vi "Unregister Event.vi"(8 "error in (no error)":errorcluster, 9 "EventToken":refnum<class "EventToken.lvclass">, 11 "ActiveObjectEventManager in":refnum<class "EventManager.lvclass">) -> (0 "error out":errorcluster, 3 "ActiveObjectEventManager out":refnum<class "EventManager.lvclass">)   [LabVIEW 2009, in "EventManagerLibrary.lvlib" / "EventManager.lvclass"]
uses:
  EventManager.lvclass
  EventToken/EventToken.lvclass
  EventManager.lvclass/EventManager.ctl
  EventBag/EventBag.lvclass
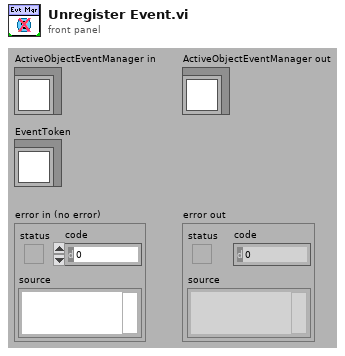
[diagram p1: front panel]
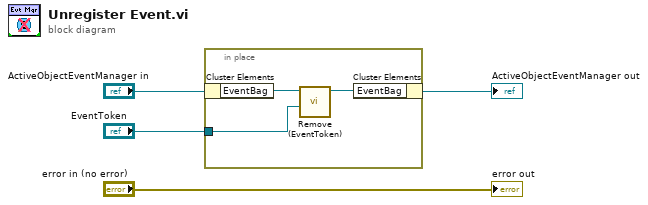
[diagram p0: block diagram]
diagram:
  n1 = in-place {
    in-place-border: "EventToken" -> [w5]
    n2 = in-place-cluster #1("ActiveObjectEventManager in") -> ("EventBag"=w7:refnum<class "EventBag.lvclass">)
    n3 = call-dynamic "Remove (EventToken).vi"("EventToken"=w5, "EventBag in"=w7) -> ("EventBag out"=w6:refnum<class "EventBag.lvclass">)  [unwired: 1 in, 8 out]
    n4 = in-place-cluster #1("EventBag"=w6) -> (→"ActiveObjectEventManager out":refnum<class "EventManager.lvclass">)
  }
  "error out" <- "error in (no error)"
